vi "Clase6.vi"() -> ()   [LabVIEW 2011]
panel:
  out "ALARMA":bool
  out "Temperatura":dbl(slide) scale=0.0..100.0
  out "Velocidad Super Rapida":bool
  out "Velocidad RAPIDA":bool
  out "Velocidad Lenta":bool
  out "Velocidad":i32(knob) scale=0.0..220.0
  # "SE TIENE QUE GENERAR LA VELOCIDAD ENTRE 1-220\n\nLUEGO SE ENCIENDEN LOS LED DE ACUERDO A LA VELOCIDAD \n1-80 LENTA\n81-120 RAPIDA\n121-220 MUY RAPIDA\n\nLUEGO SI LA TEMPERATURA ESTA ARRIBA DE LOS 75 GRADOS Y LA VELOCIDAD ES MUY\nRAPIDA SE TIENE QUE ENCENDER EL LED DE LA ALARMA."
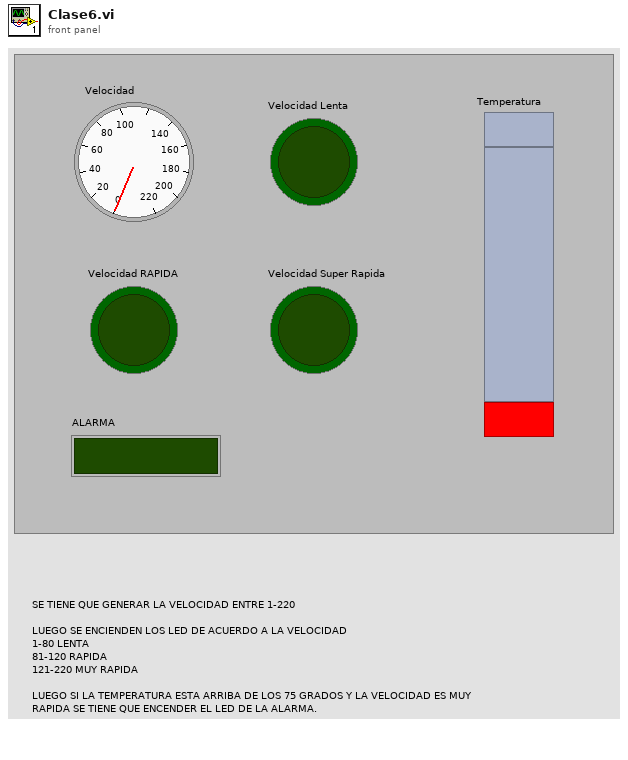
[diagram p1: front panel]
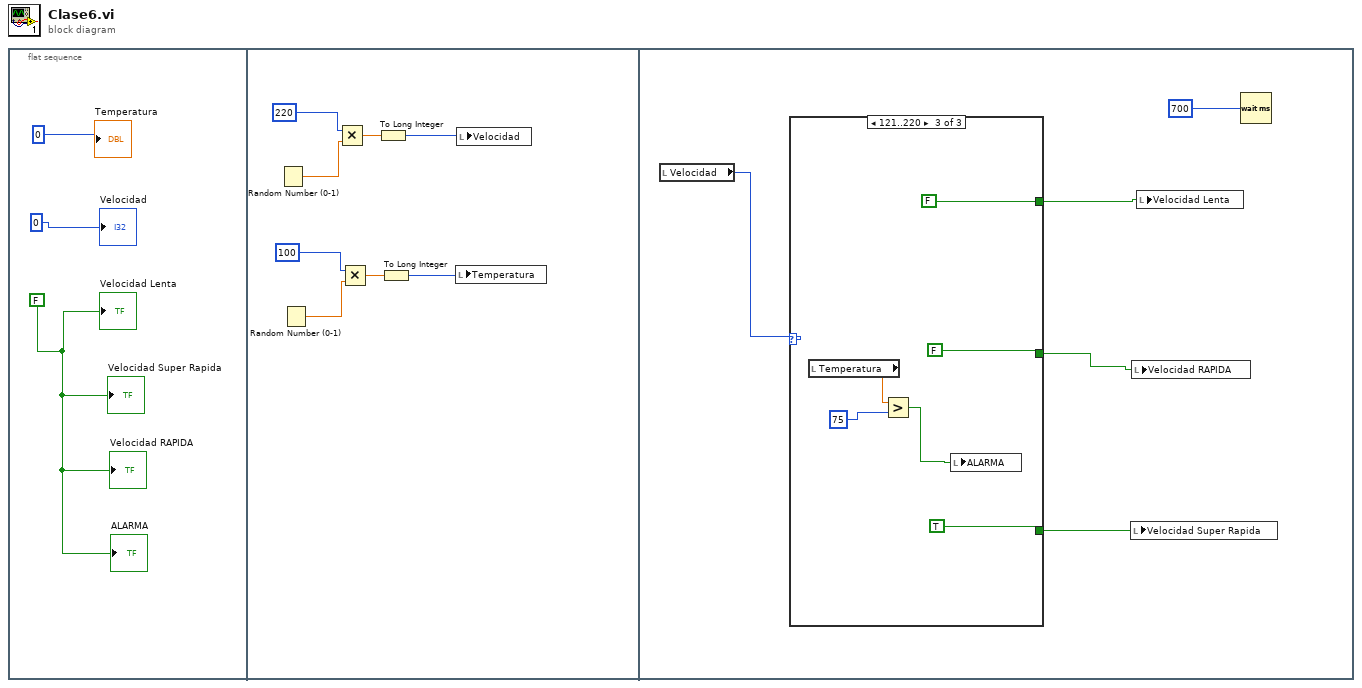
[diagram p0: block diagram]
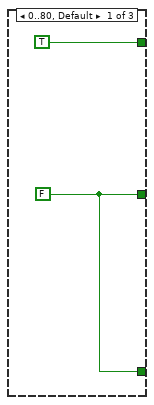
[diagram p2: hidden frame]
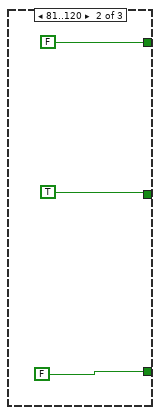
[diagram p3: hidden frame]
diagram:
  n1 = flat-sequence {
    frame #0 {
      w2 = FALSE
      "Velocidad" <- 0
      "Temperatura" <- 0
      "Velocidad Super Rapida" <- w2
      "Velocidad RAPIDA" <- w2
      "Velocidad Lenta" <- w2
      "ALARMA" <- w2
    }
    frame #1 {
      n2 = Random Number (0-1)() -> (number: 0 to 1=w11:dbl)
      n3 = Random Number (0-1)() -> (number: 0 to 1=w6:dbl)
      n4 = Multiply(x=220, y=w11) -> (x*y=w9:dbl)
      n5 = Multiply(x=100, y=w6) -> (x*y=w8:dbl)
      n6 = To Long Integer(number=w9) -> (32bit integer=w4:i32)
      n7 = To Long Integer(number=w8) -> (32bit integer=w5:i32)
      n8 = local write "Temperatura"(w5) -> ()
      n9 = local write "Velocidad"(w4) -> ()
    }
    frame #2 {
      n10 = local read "Velocidad"() -> (w16:i32)
      n11 = case shown="121..220" w16 {
        tunnel: [TRUE FALSE FALSE] -> w15
        tunnel: [w17 TRUE FALSE] -> w14
        tunnel: [w17 FALSE TRUE] -> w13
        frame 0..80, Default {
          w17 = FALSE
        }
        frame 81..120 {
        }
        frame 121..220 {
          n12 = local read "Temperatura"() -> (w25:dbl)
          n13 = Greater?(x=w25, y=75) -> (0:w23:bool)
          n14 = local write "ALARMA"(w23) -> ()
        }
      }
      n15 = local write "Velocidad Super Rapida"(w13) -> ()
      n16 = local write "Velocidad RAPIDA"(w14) -> ()
      n17 = local write "Velocidad Lenta"(w15) -> ()
      n18 = Wait (ms)(milliseconds to wait=700) -> ()  [unwired: 1 out]
    }
  }
